vi "getTestIdlFilePath.vi"() -> (3 "testIdlPath":path)   [LabVIEW 2018]
doc: "Get the test IDL file path."
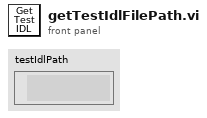
[diagram p1: front panel]
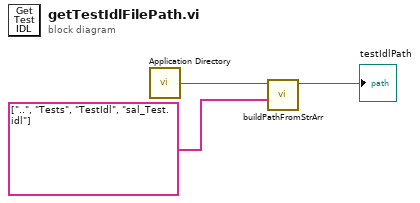
[diagram p0: block diagram]
diagram:
  n1 = call <vilib>:"Application Directory.vi"() -> ("Application Directory"=w2:path)
  n2 = call "buildPathFromStrArr.vi"("String Array"=string[] ["..", "Tests", "TestIdl", "sal_Test.idl"], "Root Path"=w2) -> ("Absolute Path"=→"testIdlPath":path)  [unwired: 9 in]
